vi "Step of Steps Params.vi"(7 "Step of STEP params":T1, 8 "error in (no error)":errorcluster, 10 "Step NO":u8=1 min=1 max=50 step=1, 11 "Profile NO":u8=1 min=1 max=50 step=1) -> (0 "error out":errorcluster, 2 "wchitch params":string, 3 "params array out":string[](array[string]))   [LabVIEW 2019, in "STAV lib.lvlib"]
uses:
  STAV lib.lvlib
  Step of Step params.ctl
  Param Direction.ctl
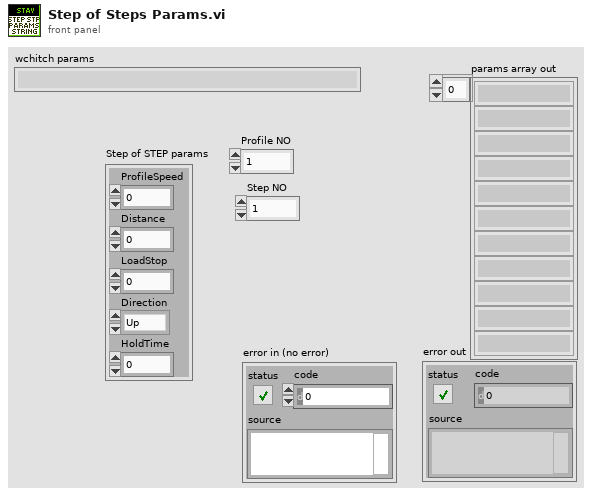
[diagram p1: front panel]
types:
  T1 = typedef "STAV lib.lvlib/Step of Step params.ctl" = cluster{"ProfileSpeed":dbl, "Distance":dbl, "LoadStop":dbl, "Direction":T2, "HoldTime":dbl}
  T2 = typedef "STAV lib.lvlib/Param Direction.ctl" = enum16{"Up", "Down", "Left", "Right"}
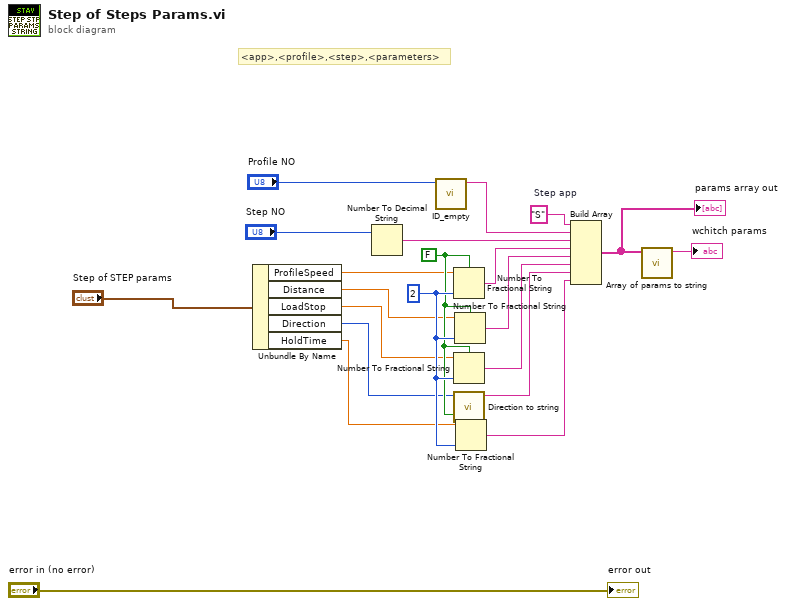
[diagram p0: block diagram]
diagram:
  w18 = i16 2 ("precision (6)")
  w17 = FALSE ("use system decimal point (T)")
  w1 = "S"  # Step app
  # "<app>,<profile>,<step>,<parameters>"
  n1 = Unbundle By Name("Step of STEP params") -> ("ProfileSpeed"=w11:dbl, "Distance"=w10:dbl, "LoadStop"=w9:dbl, "Direction"=w5:T2, "HoldTime"=w8:dbl)
  n2 = Number To Decimal String(number="Step NO") -> (decimal integer string=w3:string)  [unwired: 1 in]
  n3 = call "ID_empty.vi"("Profile NO"="Profile NO") -> ("Profile NO out"=w2:string)  [unwired: 9 in, 1 out]
  n4 = Number To Fractional String(use system decimal point (T)=w17, number=w11, precision (6)=w18) -> (F-format string=w19:string)  [unwired: 1 in]
  n5 = Number To Fractional String(use system decimal point (T)=w17, number=w9, precision (6)=w18) -> (F-format string=w15:string)  [unwired: 1 in]
  n6 = call "Direction to string.vi"("Direction"=w5) -> ("Peak app"=w6:string)  [unwired: 10 in]
  n7 = Number To Fractional String(use system decimal point (T)=w17, number=w10, precision (6)=w18) -> (F-format string=w16:string)  [unwired: 1 in]
  n8 = Number To Fractional String(use system decimal point (T)=w17, number=w8, precision (6)=w18) -> (F-format string=w7:string)  [unwired: 1 in]
  n9 = Build Array(w1, w2, w3, w19, w16, w15, w6, w7) -> (w14:string[])
  "params array out" <- w14
  n10 = call "Array of params to string.vi"("Array"=w14) -> ("String"=→"wchitch params":string)  [unwired: 10 in]
  "error out" <- "error in (no error)"
